vi "Teleop.vi"(10 "Match Info":T2={"Autonomous Elapsed Seconds"=0.0, "TeleOp Elapsed Seconds"=0.0, "Disabled Elapsed Seconds"=0.0, "Visited Autonomous"=FALSE, "Visited TeleOp"=FALSE, "Visited Disabled"=FALSE, "Autonomous Settings"={"Autonomous Style"=enum."Independent", "VI Refnum"=refnum}}, 11 "Call Context":T3) -> ()   [LabVIEW 2015]
doc: "This VI is called for each TeleOp packet received from the DS where the robot is not disabled. It is often used to read from the joysticks and update I/O or to update setpoints for timed control loops. It should complete and return within 20 milliseconds or it may miss DS packets."
uses:
  <vilib>/Rock Robotics/Network Tables/NT Write Numeric Array.vi
  <vilib>/Rock Robotics/Network Tables/NT Write Boolean Array.vi
  <vilib>/Rock Robotics/Network Tables/NT Read Boolean.vi
  <vilib>/Rock Robotics/Network Tables/NT Read Number.vi
  <vilib>/Rock Robotics/Network Tables/NT Write Boolean.vi
  <vilib>/Rock Robotics/Network Tables/NT Write Number.vi
  <vilib>/Rock Robotics/WPI/RobotDrive/WPI_RobotDriveArcadeDrive_Standard(NoSaturation).vi
  <vilib>/Rock Robotics/WPI/DriverStation/WPI_DriverStationMatch Info.ctl
  <vilib>/Rock Robotics/WPI/DriverStation/WPI_DriverStationDerivedRobotMode.ctl
panel:
  out "ElevatorENC RATE":dbl(graph)
  out "ElevatorENC DIST":dbl(graph)
  in  "PID gains 2":T1={"proportional gain (Kc)"=1.0, "integral time (Ti, min)"=0.01, "derivative time (Td, min)"=0.0} {"derivative time (Td, min)" format="%.3f"; "integral time (Ti, min)" format="%.3f"; "proportional gain (Kc)" format="%.3f"}
  out "Right Drive Sped":dbl(graph)
  out "Left Drive Sped":dbl(graph)
  out "Right Drive Dist":dbl(graph)
  out "Left Drive Dist":dbl(graph)
  in  "Lower Limit":dbl
  in  "Upper Limit":dbl=4.0
  out "Sample Slider 0":dbl(slide) scale=0.0..5.0
  out "Sample Boolean 1":bool
  out "Sample Boolean 0":bool
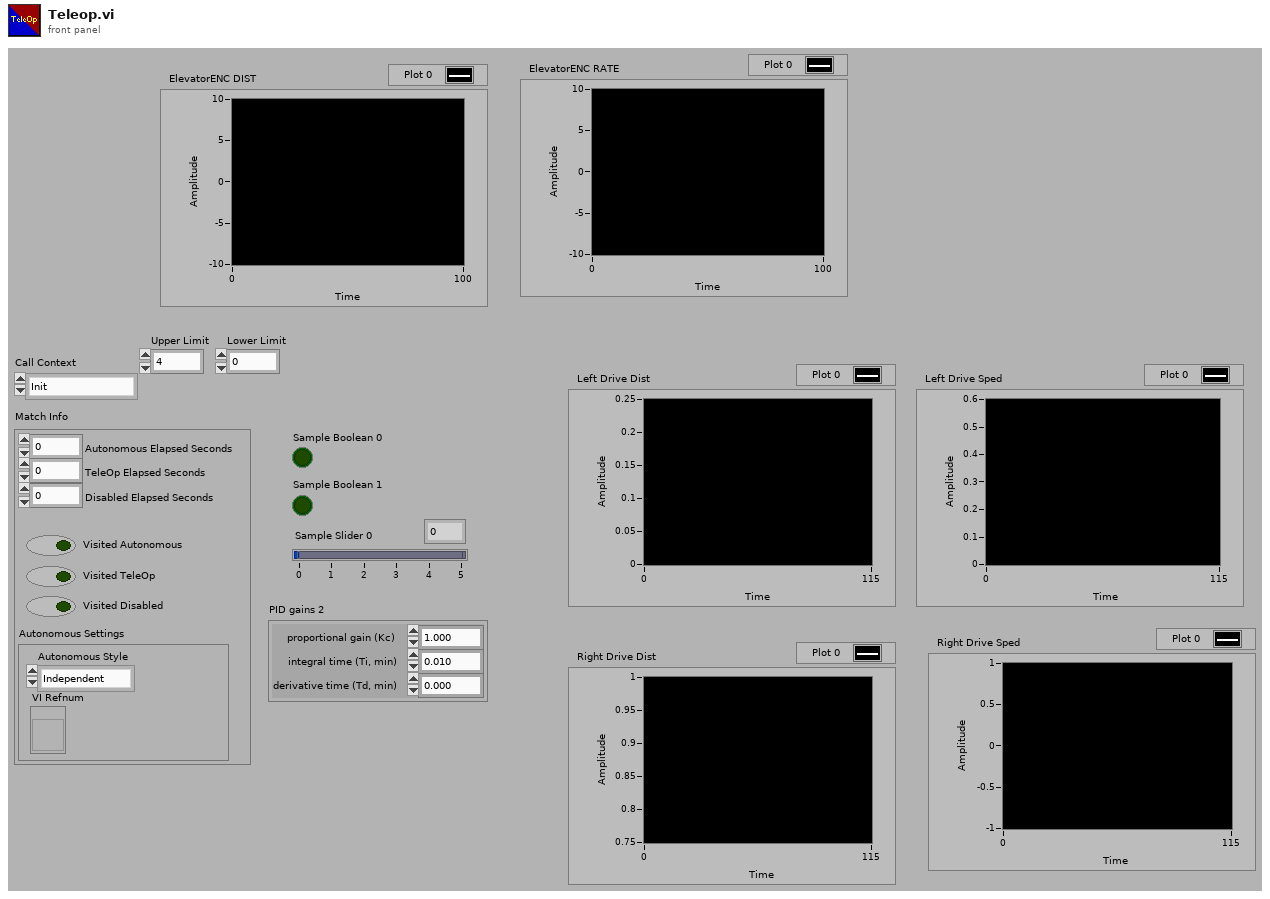
[diagram p1: front panel]
types:
  T1 = cluster{"proportional gain (Kc)":dbl, "integral time (Ti, min)":dbl, "derivative time (Td, min)":dbl}
  T2 = typedef "WPI_DriverStationMatch Info.ctl" = cluster{"Autonomous Elapsed Seconds":dbl, "TeleOp Elapsed Seconds":dbl, "Disabled Elapsed Seconds":dbl, "Visited Autonomous":bool, "Visited TeleOp":bool, "Visited Disabled":bool, "Autonomous Settings":cluster{"Autonomous Style":enum16{"Iterative", "Independent"}, "VI Refnum":refnum<vi>}}
  T3 = typedef "WPI_DriverStationDerivedRobotMode.ctl" = enum16{"Init", "Execute", "Stop"}
  T4 = typedef "WPI_GyroDevRef.ctl" = cluster{"DevStatus":errorcluster, "Analog Channel":T5, "Offset":dbl, "Gain (VoltsPerDegree/Second)":dbl, "Gyro Type":enum16{"Analog", "XRS450"}, "Handle":i32, "SPI Bus":T6, "Device Found":bool, "Sample Rate":dbl, "Calibrate On Open":bool}
  T5 = typedef "FPGA_AIChannel.ctl" = enum8{"AI 0", "AI 1", "AI 2", "AI 3", "AI MXP 0", "AI MXP 1", "AI MXP 2", "AI MXP 3", "Invalid"}
  T6 = typedef "spi_bus.ctl" = enum16{"SPI On-Board, CS0", "SPI On-Board, CS1", "SPI On-Board, CS2", "SPI On-Board, CS3", "SPI MXP", "Invalid"}
  T7 = typedef "WPI_EncoderDevRef.ctl" = cluster{"DevStatus":errorcluster, "EncoderIndex":T8, "CounterIndex":T9, "DistancePerCount":dbl, "Decoding Type":T10}
  T8 = typedef "FPGA_EncoderIdx.ctl" = enum8{"Enc 0", "Enc 1", "Enc 2", "Enc 3", "Enc 4", "Enc 5", "Enc 6", "Enc 7", "Invalid"}
  T9 = typedef "FPGA_CounterCtrSystemIndex.ctl" = enum8{"Ctr 0", "Ctr 1", "Ctr 2", "Ctr 3", "Ctr 4", "Ctr 5", "Ctr 6", "Ctr 7", "Invalid"}
  T10 = typedef "WPI_EncoderType.ctl" = enum16{"1x", "2x", "4x"}
  T11 = typedef "WPI_JoystickDevRef.ctl" = cluster{"Device":T12}
  T12 = typedef "WPI_JoystickDeviceEnum.ctl" = enum16{"USB 0", "USB 1", "USB 2", "USB 3", "USB 4", "USB 5"}
  T13 = typedef "WPI_MotorControlDeviceRef.ctl" = cluster{"DeviceStatus":errorcluster, "Type":T14, "PWM":cluster{"PWM Channel":T15, "DeadBand":T16}, "CAN":cluster{"Device Number":u8, "Control Mode":T17, "Semaphore":T18, "Max Vout":dbl, "TalonSRX Control Mode":T19}, "Invert":bool}
  T14 = typedef "WPI_MotorControlType.ctl" = enum16{"PWM", "CAN", "CANTalonSRX"}
  T15 = typedef "FPGA_DIOPWMChannel.ctl" = enum8{"PWM 0", "PWM 1", "PWM 2", "PWM 3", "PWM 4", "PWM 5", "PWM 6", "PWM 7", "PWM 8", "PWM 9", "PWM MXP 0", "PWM MXP 1", "PWM MXP 2", "PWM MXP 3", "PWM MXP 4", "PWM MXP 5", "PWM MXP 6", "PWM MXP 7", "PWM MXP 8", "PWM MXP 9", "Invalid"}
  T16 = typedef "WPI_PWMDeadband.ctl" = cluster{"Name":string, "maxPositivePwm":i32, "minPositivePwm":i32, "centerPwm":i32, "maxNegativePwm":i32, "minNegativePwm":i32, "angularRange":u16}
  T17 = typedef "WPI_CANJaguar_ControlMode.ctl" = enum8{"Percent VBus", "Current", "Speed", "Position", "Voltage"}
  T18 = typedef "Semaphore RefNum" = refnum<k1>
  T19 = typedef "WPI_CANTalonSRX_APIControlMode.ctl" = enum8{"Percent VBus", "Speed", "Position", "Slave", "Unchanged / Invalid", "Voltage Compensation", "Current", "Motion Profile"}
  T20 = typedef "WPI_RobotDriveDevRef.ctl" = cluster{"DevStatus":errorcluster, "Motors[]":T13[], "Square Inputs":bool, "Max Output":dbl}
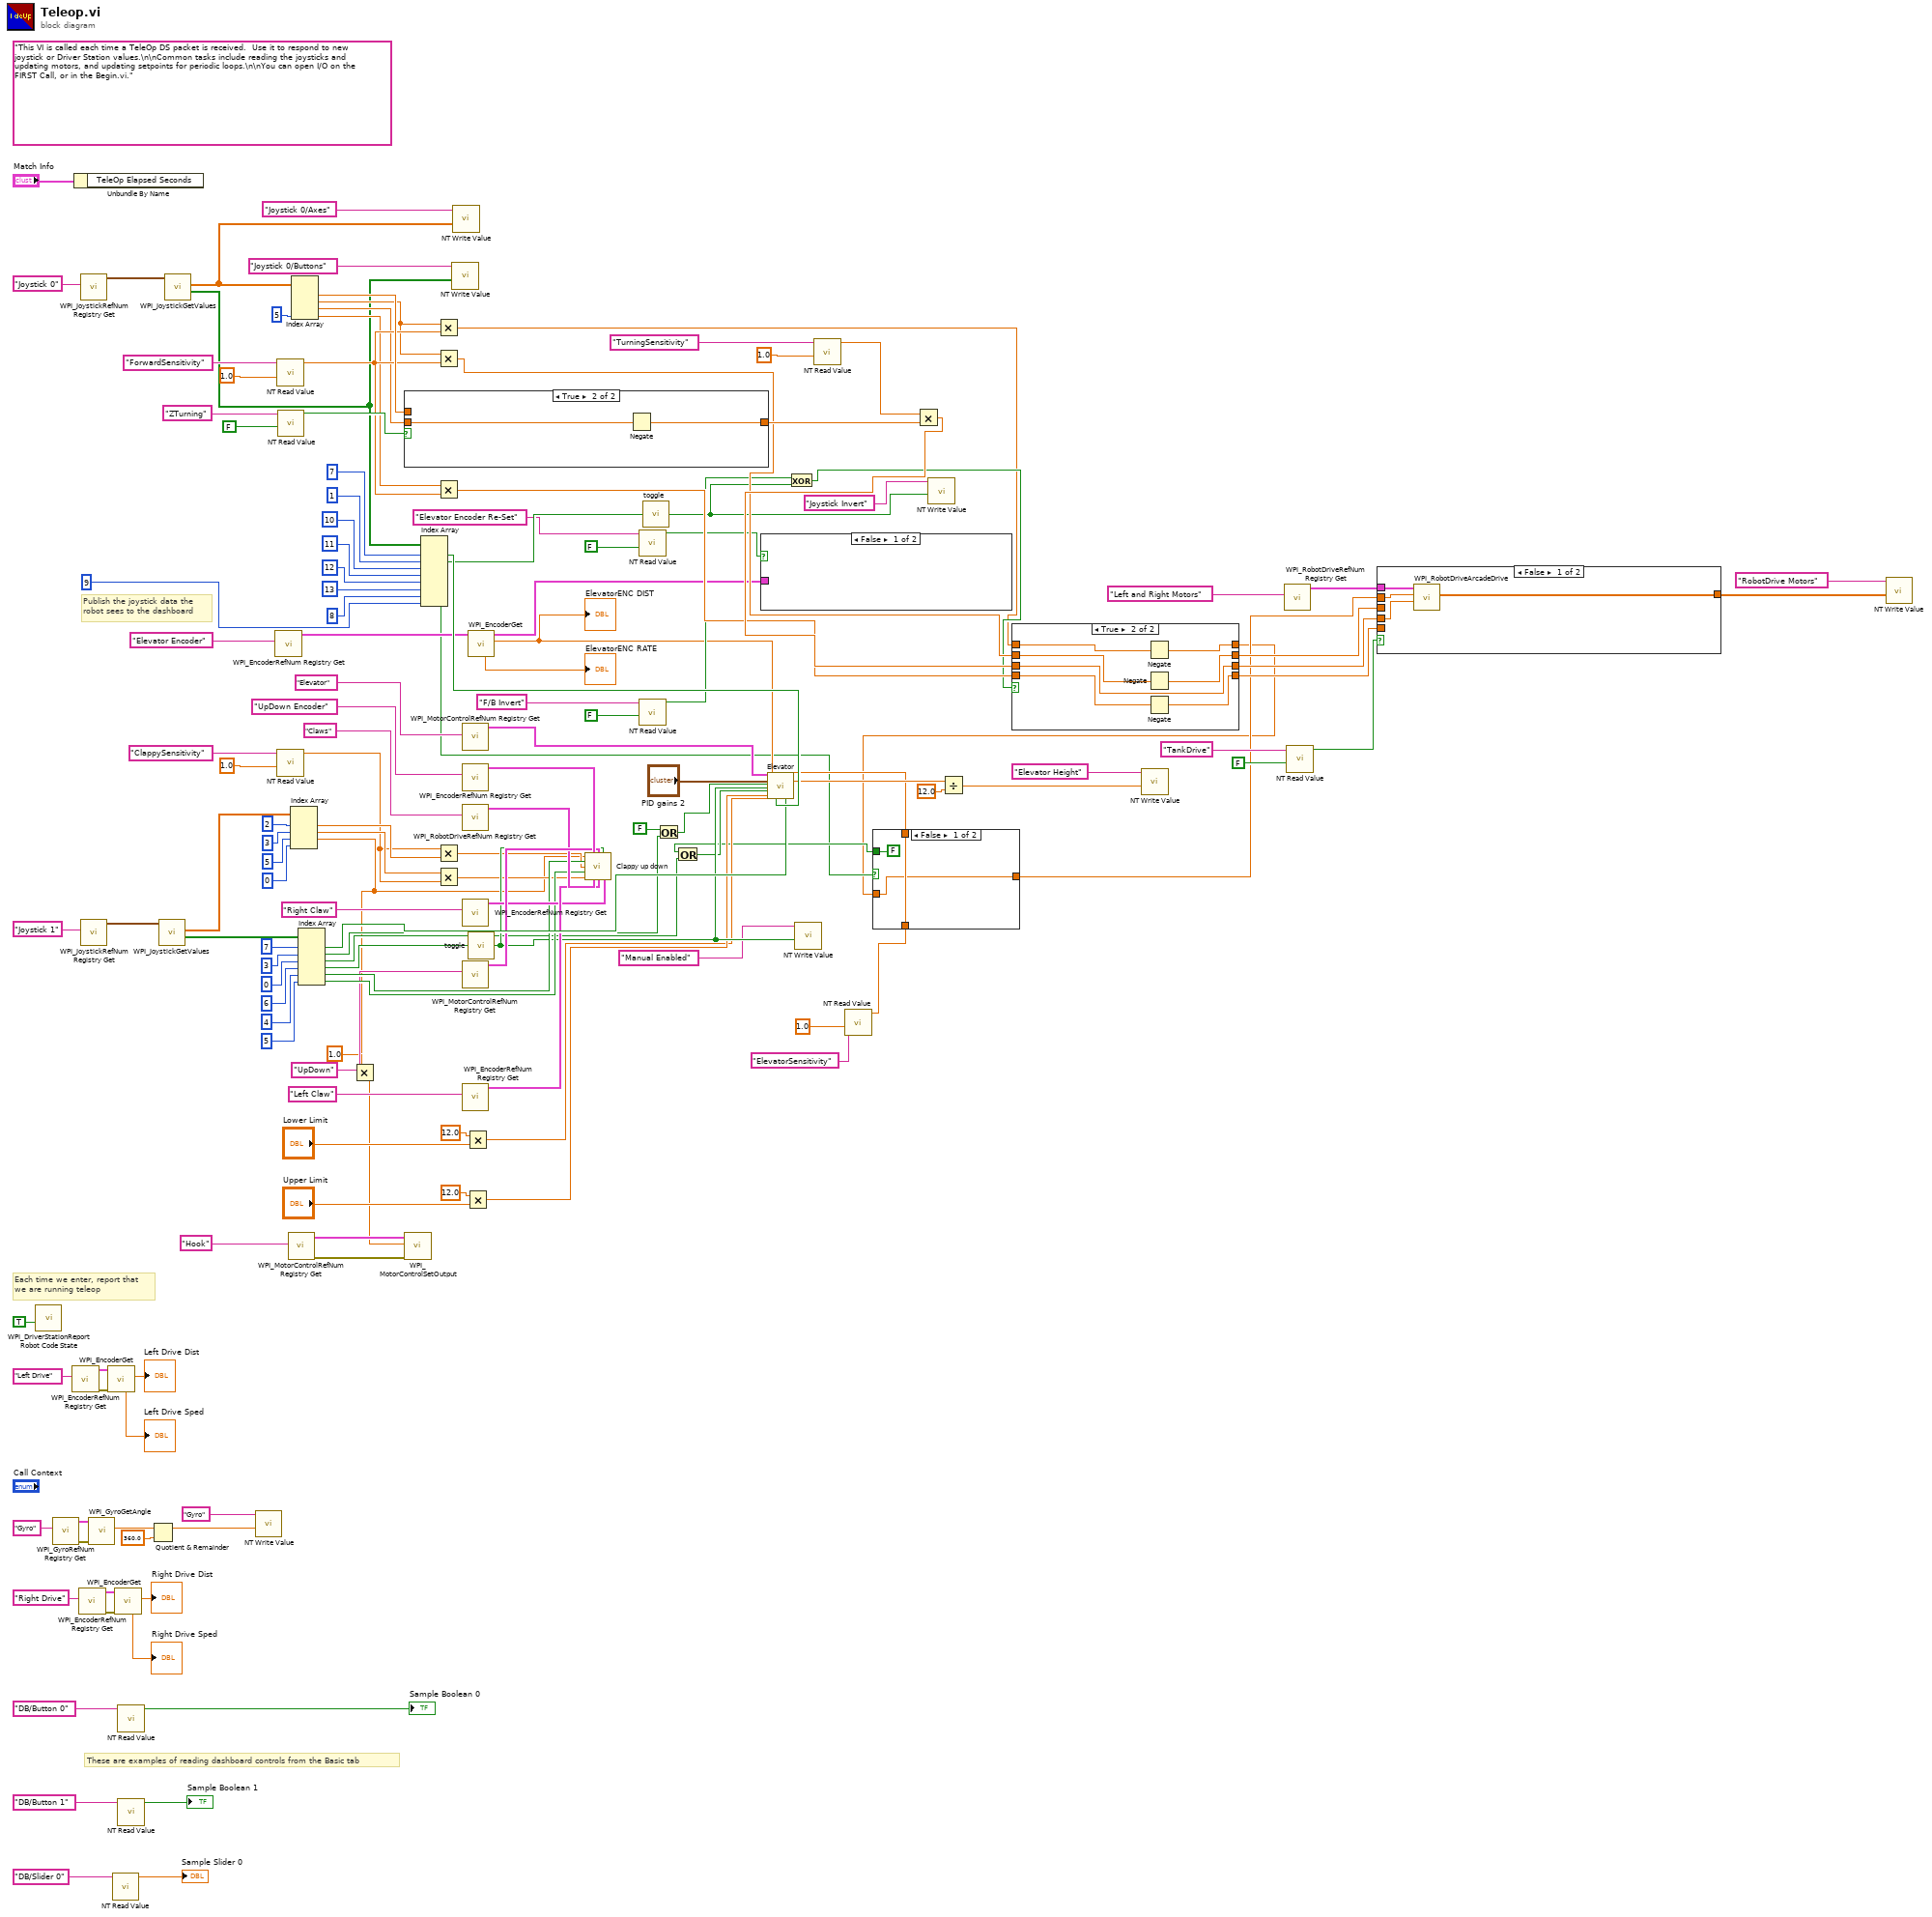
[diagram p0: block diagram]
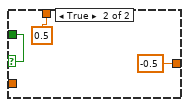
[diagram p2: hidden frame]
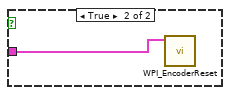
[diagram p3: hidden frame]
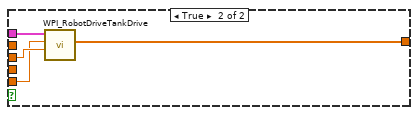
[diagram p5: hidden frame]
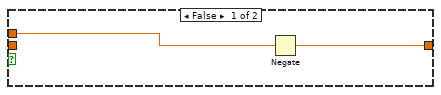
[diagram p6: hidden frame]
diagram:
  (unwired) "This VI is called each time a TeleOp DS packet is received.  Use it to respond to new joystick or Driver Station values.\n\nCommon tasks include reading the joysticks and updating motors, and updating setpoints for periodic loops.\n\nYou can open I/O on the FIRST Call, or in the Begin.vi."
  # "These are examples of reading dashboard controls from the Basic tab"
  # "Publish the joystick data the\nrobot sees to the dashboard"
  # "Each time we enter, report that\nwe are running teleop"
  n1 = call <vilib>:"WPI_DriverStationReport Robot Code State.vi"("TeleOp"=TRUE ("Autonomous")) -> ()  [unwired: 10 in, 1 out]
  n2 = call <vilib>:"WPI_GyroRefNum Registry Get.vi"("refnum name"="Gyro") -> ("error out"=w59:errorcluster, "GyroDevRef"=w60:T4)  [unwired: 9 in]
  n3 = call <vilib>:"WPI_EncoderRefNum Registry Get.vi"("refnum name"="Left Drive") -> ("error out"=w72:errorcluster, "EncoderDevRef"=w71:T7)  [unwired: 9 in]
  n4 = Unbundle By Name("Match Info") -> ()  [unwired: 1 out]
  n5 = call <vilib>:"WPI_EncoderRefNum Registry Get.vi"("refnum name"="Right Drive") -> ("error out"=w70:errorcluster, "EncoderDevRef"=w69:T7)  [unwired: 9 in]
  n6 = call <vilib>:"WPI_JoystickRefNum Registry Get.vi"("refnum name"="Joystick 0") -> ("JoystickDevRef"=w149:T11)  [unwired: 1 in, 9 out]
  n7 = call <vilib>:"WPI_JoystickRefNum Registry Get.vi"("refnum name"="Joystick 1") -> ("JoystickDevRef"=w114:T11)  [unwired: 1 in, 9 out]
  n8 = call <vilib>:"WPI_GyroGetAngle.vi"("error in"=w59, "GyroDevRef"=w60) -> ("Angle"=w55:dbl)  [unwired: 5 in, 4 out]
  n9 = call <vilib>:"WPI_EncoderGet.vi"("error in (no error)"=w72, "EncoderDevRef"=w71) -> ("Distance"=→"Left Drive Dist":dbl, "Rate"=→"Left Drive Sped":dbl)  [unwired: 4 in, 4 out]
  n10 = call-poly <vilib>:"NT Read Value.vi"("Name"="DB/Slider 0" ("refnum name")) -> ("Numeric"=→"Sample Slider 0":dbl)  [unwired: 9 in, 1 out]
  n11 = call <vilib>:"WPI_EncoderGet.vi"("error in (no error)"=w70, "EncoderDevRef"=w69) -> ("Distance"=→"Right Drive Dist":dbl, "Rate"=→"Right Drive Sped":dbl)  [unwired: 4 in, 4 out]
  n12 = call-poly <vilib>:"NT Read Value.vi"("Name"="DB/Button 0" ("refnum name")) -> ("Boolean"=→"Sample Boolean 0":bool)  [unwired: 9 in, 1 out]
  n13 = call-poly <vilib>:"NT Read Value.vi"("Name"="DB/Button 1" ("refnum name")) -> ("Boolean"=→"Sample Boolean 1":bool)  [unwired: 9 in, 1 out]
  n14 = Quotient & Remainder(x=w55, y=360.0) -> (x-y*floor(x/y)=w54:dbl)  [unwired: 1 out]
  n15 = call <vilib>:"WPI_JoystickGetValues.vi"("JoystickDevRef"=w114) -> ("Buttons"=w113:bool[], "Axes"=w100:dbl[])  [unwired: 6 in, 3 out]
  n16 = call <vilib>:"WPI_JoystickGetValues.vi"("JoystickDevRef"=w149) -> ("Buttons"=w118:bool[], "Axes"=w145:dbl[])  [unwired: 6 in, 3 out]
  n17 = call-poly <vilib>:"NT Write Value.vi"("Numeric"=w54, "Name"="Gyro") -> ()  [unwired: 9 in, 1 out]
  n18 = call <vilib>:"WPI_EncoderRefNum Registry Get.vi"("refnum name"="Elevator Encoder") -> ("EncoderDevRef"=w44:T7)  [unwired: 9 in, 1 out]
  n19 = call-poly <vilib>:"NT Read Value.vi"("Default Value"=1.0, "Name"="ForwardSensitivity") -> ("Numeric"=w127:dbl)  [unwired: 8 in, 1 out]
  n20 = call-poly <vilib>:"NT Read Value.vi"("Default Value"=1.0, "Name"="ClappySensitivity") -> ("Numeric"=w20:dbl)  [unwired: 8 in, 1 out]
  n21 = call-poly <vilib>:"NT Read Value.vi"("Default Value"=FALSE, "Name"="ZTurning") -> ("Boolean"=w134:bool)  [unwired: 8 in, 1 out]
  n22 = call <vilib>:"WPI_MotorControlRefNum Registry Get.vi"("refnum name"="Hook") -> ("error out"=w27:errorcluster, "MotorControlDevRef"=w26:T13)  [unwired: 9 in]
  n23 = Index Array(array=w100, index #1=2 ("index"), index #2=3 ("index"), index #3=5 ("index"), index #4=0 ("index")) -> (element #1=w93:dbl, element #2=w92:dbl, element #3=w1:dbl)  [unwired: 1 out]
  n24 = Index Array(array=w145, index #4=5 ("index")) -> (element #1=w128:dbl, element #2=w122:dbl, element #3=w120:dbl, element #4=w119:dbl)  [unwired: 3 in]
  n25 = Index Array(array=w113, index #1=7 ("index"), index #2=3 ("index"), index #3=0 ("index"), index #4=6 ("index"), index #5=4 ("index"), index #6=5 ("index")) -> (element #1=w111:bool, element #2=w15:bool, element #3=w13:bool, element #4=w102:bool, element #5=w90:bool, element #6=w89:bool)
  n26 = Multiply(x=w1, y=1.0) -> (x*y=w3:dbl)
  n27 = case shown="True" w134 {
    tunnel: w120 -> [_ w156]
    tunnel: [w154 w157] -> w124
    tunnel: w128 -> [w155 _]
    frame False {
      n28 = Negate(x=w155) -> (-x=w154:dbl)
    }
    frame True {
      n29 = Negate(x=w156) -> (-x=w157:dbl)
    }
  }
  n30 = call <vilib>:"WPI_MotorControlSetOutput.vi"("error in (no error)"=w27, "Output"=w3, "MotorControlDevRef"=w26) -> ()  [unwired: 6 in, 3 out]
  n31 = Index Array(array=w118, index #1=7 ("index"), index #2=1 ("index"), index #3=10 ("index"), index #4=11 ("index"), index #5=12 ("index"), index #6=13 ("index"), index #7=8 ("index"), index #8=9 ("index")) -> (element #1=w116:bool, element #2=w77:bool, element #8=w6:bool)  [unwired: 5 out]
  n32 = Multiply(x=w122, y=w127) -> (x*y=w18:dbl)
  n33 = Multiply(x=w122, y=w127) -> (x*y=w84:dbl)
  n34 = Multiply(x=w119, y=w127) -> (x*y=w82:dbl)
  n35 = Multiply(x=w20, y=w93) -> (x*y=w24:dbl)
  n36 = Multiply(x=w92, y=w20) -> (x*y=w23:dbl)
  n37 = call-poly <vilib>:"NT Write Value.vi"("Boolean Array"=w118, "Name"="Joystick 0/Buttons") -> ()  [unwired: 9 in, 1 out]
  n38 = call-poly <vilib>:"NT Write Value.vi"("Numeric Array"=w145, "Name"="Joystick 0/Axes") -> ()  [unwired: 9 in, 1 out]
  n39 = call <vilib>:"WPI_MotorControlRefNum Registry Get.vi"("refnum name"="Elevator") -> ("MotorControlDevRef"=w47:T13)  [unwired: 9 in, 1 out]
  n40 = call <vilib>:"WPI_EncoderRefNum Registry Get.vi"("refnum name"="UpDown Encoder") -> ("EncoderDevRef"=w101:T7)  [unwired: 9 in, 1 out]
  n41 = call <vilib>:"WPI_RobotDriveRefNum Registry Get.vi"("refnum name"="Claws") -> ("RobotDriveDevRef"=w96:T20)  [unwired: 9 in, 1 out]
  n42 = call <vilib>:"WPI_EncoderRefNum Registry Get.vi"("refnum name"="Right Claw") -> ("EncoderDevRef"=w94:T7)  [unwired: 9 in, 1 out]
  n43 = call <vilib>:"WPI_MotorControlRefNum Registry Get.vi"("refnum name"="UpDown") -> ("MotorControlDevRef"=w97:T13)  [unwired: 9 in, 1 out]
  n44 = call <vilib>:"WPI_EncoderRefNum Registry Get.vi"("refnum name"="Left Claw") -> ("EncoderDevRef"=w95:T7)  [unwired: 9 in, 1 out]
  n45 = Multiply(x=12.0, y="Lower Limit") -> (x*y=w37:dbl)
  n46 = Multiply(x=12.0, y="Upper Limit") -> (x*y=w39:dbl)
  n47 = call <vilib>:"WPI_EncoderGet.vi"("EncoderDevRef"=w44) -> ("Distance"=w19:dbl, "EncoderDevRef"=w32:T7, "Rate"=→"ElevatorENC RATE":dbl)  [unwired: 5 in, 3 out]
  "ElevatorENC DIST" <- w19
  n48 = call "toggle.vi"("Input"=w102) -> ("Output"=w63:bool)
  n49 = call "Clappy up down.vi"("UP/Down"=w1, "UP DOWN ENCODER"=w101, "UPDOWN"=w97, "Manual"=w63, "Negate 1"=w90, "Open/Closed 1"=w24, "Negate 2"=w89, "Open/Closed 2"=w23, "Clappy"=w96, "OPEN CLOSED ENCODER 1"=w95, "OPEN CLOSED ENCODER 2"=w94) -> ()  [unwired: 5 in]
  n50 = call-poly <vilib>:"NT Read Value.vi"("Default Value"=FALSE, "Name"="Elevator Encoder Re-Set") -> ("Boolean"=w29:bool)  [unwired: 8 in, 1 out]
  n51 = call-poly <vilib>:"NT Read Value.vi"("Default Value"=FALSE, "Name"="F/B Invert") -> ("Boolean"=w79:bool)  [unwired: 8 in, 1 out]
  n52 = call "toggle.vi"("Input"=w77) -> ("Output"=w76:bool)
  n53 = Or(x=FALSE, y=w15) -> (x .or. y?=w16:bool)
  n54 = case shown="False" w29 {
    tunnel: w32 -> [_ w158]
    frame False {
    }
    frame True {
      n55 = call <vilib>:"WPI_EncoderReset.vi"("EncoderDevRef"=w158) -> ()  [unwired: 9 in, 2 out]
    }
  }
  n56 = Exclusive Or(1:w76, 2:w79) -> (0:w78:bool)
  n57 = call-poly <vilib>:"NT Write Value.vi"("Boolean"=w63, "Name"="Manual Enabled") -> ()  [unwired: 9 in, 1 out]
  n58 = call-poly <vilib>:"NT Read Value.vi"("Default Value"=1.0, "Name"="TurningSensitivity") -> ("Numeric"=w123:dbl)  [unwired: 8 in, 1 out]
  n59 = call-poly <vilib>:"NT Read Value.vi"("Default Value"=1.0, "Name"="ElevatorSensitivity") -> ("Numeric"=w9:dbl)  [unwired: 8 in, 1 out]
  n60 = Multiply(x=w123, y=w124) -> (x*y=w86:dbl)
  n61 = call-poly <vilib>:"NT Write Value.vi"("Boolean"=w76, "Name"="Joystick Invert") -> ()  [unwired: 9 in, 1 out]
  n62 = case shown="True" w78 {
    tunnel: [w162 w163] -> w87
    tunnel: w86 -> [w162 w163]
    tunnel: [w161 w169] -> w85
    tunnel: w84 -> [w161 w168]
    tunnel: [w160 w166] -> w4
    tunnel: w18 -> [w160 w167]
    tunnel: [w159 w164] -> w83
    tunnel: w82 -> [w159 w165]
    frame False {
    }
    frame True {
      n63 = Negate(x=w167) -> (-x=w166:dbl)
      n64 = Negate(x=w168) -> (-x=w169:dbl)
      n65 = Negate(x=w165) -> (-x=w164:dbl)
    }
  }
  n66 = case shown="False" w6 {
    selector: w6 -> [_ w174]
    tunnel: [w172 0.5 ("Numeric")] -> w10
    tunnel: w9 -> [w172 _]
    tunnel: [FALSE w174] -> w7
    tunnel: [w170 -0.5] -> w5
    tunnel: w4 -> [w170 _]
    frame False {
    }
    frame True {
    }
  }
  n67 = Or(x=w7, y=w13) -> (x .or. y?=w14:bool)
  n68 = call "Elevator.vi"("MotorControlDevRef"=w47, "PID gains"="PID gains 2", "Upper"=w16, "Manual"=w63, "Lower"=w14, "Upper Limit"=w39, "Lower Limit"=w37, "Distance"=w19, "Override Pilot"=w116, "ELEV SEMSITIVITY"=w10, "Override CoPilot"=w111) -> ("Height"=w34:dbl)  [unwired: 16 in]
  n69 = Divide(x=w34, y=12.0) -> (x/y=w35:dbl)
  n70 = call-poly <vilib>:"NT Write Value.vi"("Numeric"=w35, "Name"="Elevator Height") -> ()  [unwired: 9 in, 1 out]
  n71 = call <vilib>:"WPI_RobotDriveRefNum Registry Get.vi"("refnum name"="Left and Right Motors") -> ("RobotDriveDevRef"=w151:T20)  [unwired: 1 in, 9 out]
  n72 = call-poly <vilib>:"NT Read Value.vi"("Default Value"=FALSE, "Name"="TankDrive") -> ("Boolean"=w131:bool)  [unwired: 8 in, 1 out]
  n73 = case shown="False" w131 {
    tunnel: w151 -> [w179 w183]
    tunnel: [w178 w182] -> w138
    tunnel: w5 -> [w177 _]
    tunnel: w87 -> [w176 _]
    tunnel: w85 -> [_ w181]
    tunnel: w83 -> [_ w180]
    frame False {
      n74 = call-poly <vilib>:"WPI_RobotDriveArcadeDrive.vi"("Y axis value"=w176, "X axis value"=w177, "RobotDriveDevRef"=w179) -> ("Motor Values"=w178:dbl[])  [unwired: 6 in, 2 out]
    }
    frame True {
      n75 = call <vilib>:"WPI_RobotDriveTankDrive.vi"("Right axis value"=w181, "Left axis value"=w180, "RobotDriveDevRef"=w183) -> ("Motor Values"=w182:dbl[])  [unwired: 6 in, 2 out]
    }
  }
  n76 = call-poly <vilib>:"NT Write Value.vi"("Numeric Array"=w138, "Name"="RobotDrive Motors") -> ()  [unwired: 9 in, 1 out]
